vi "read_inverter (SubVI).vi"(8 "error in (no error)":errorcluster, 11 "Modbus Master in":refnum<class "Modbus Master.lvclass">) -> (0 "error out":errorcluster, 2 "Inverter kW":dbl, 3 "Modbus Master out":refnum<class "Modbus Master.lvclass">)   [LabVIEW 2024, in "SALICRU_MODBUS.lvlib"]
uses:
  <vilib>/Modbus/master/Modbus Master.lvclass
  SALICRU_MODBUS.lvlib
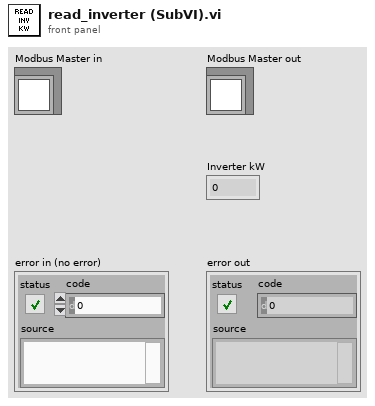
[diagram p1: front panel]
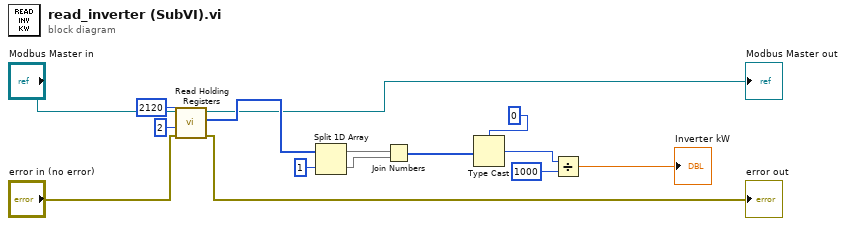
[diagram p0: block diagram]
diagram:
  n1 = call-dynamic "Read Holding Registers.vi"("error in (no error)"="error in (no error)", "number of holding registers"=u16 2, "starting address"=u16 2120, "Modbus master in"="Modbus Master in") -> ("error out"=→"error out":errorcluster, "register values"=w5:u16[], "Modbus master out"=→"Modbus Master out":refnum<class "Modbus Master.lvclass">)  [unwired: 5 in]
  n2 = Split 1D Array(array=w5, index=1) -> (first subarray=w7:u16[], second subarray=w8:u16[])
  n3 = Join Numbers(hi=w7, lo=w8) -> ((hi.lo)=w9:u32[])
  n4 = Type Cast(type=0, x=w9) -> (*(type *) &x=w13:i32)
  n5 = Divide(x=w13, y=1000) -> (x/y=→"Inverter kW":dbl)
